vi "Transmit CAN.vi"(0 "CAN Queue":T1, 2 "CAN frame":T2 {"type" items=["CAN Data", "CAN Remote"]; "identifier" format="%.0x"}) -> (7 "CAN Queue Out":T1)   [LabVIEW 2014]
uses:
  <vilib>/RioEmbeddedCAN/RioEmbeddedCAN.llb/CANFrameControl.ctl
  CAN Message Queue.ctl
  CAN Message.ctl
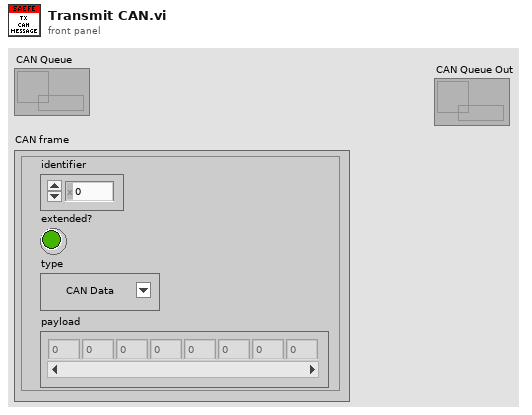
[diagram p1: front panel]
types:
  T1 = typedef "CAN Message Queue.ctl" = refnum<k33>
  T2 = typedef "CANFrameControl.ctl" = cluster{"identifier":u32, "extended?":bool, "type":u8, "payload":u8[]}
  T3 = cluster{"B0":u8, "B1":u8, "B2":u8, "B3":u8, "B4":u8, "B5":u8, "B6":u8, "B7":u8}
  T4 = typedef "CAN Message.ctl" = cluster{"identifier":u32, "extended?":bool, "type":u8, "data":cluster{"B0":u8, "B1":u8, "B2":u8, "B3":u8, "B4":u8, "B5":u8, "B6":u8, "B7":u8}}
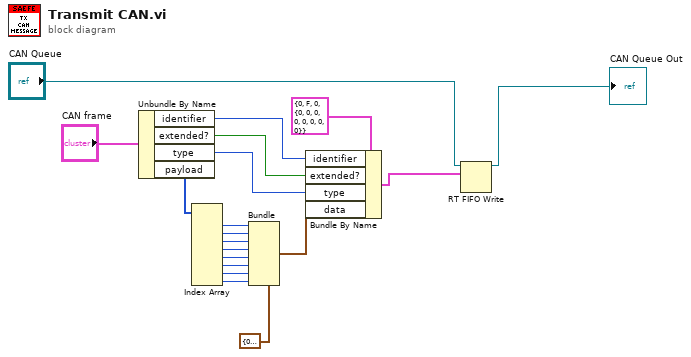
[diagram p0: block diagram]
diagram:
  n1 = Unbundle By Name("CAN frame") -> ("identifier"=w15:u32, "extended?"=w14:bool, "type"=w13:u8, "payload"=w12:u8[])
  n2 = Index Array(array=w12) -> (element #1=w11:u8, element #2=w10:u8, element #3=w9:u8, element #4=w8:u8, element #5=w7:u8, element #6=w6:u8, element #7=w5:u8, element #8=w4:u8)  [unwired: 8 in]
  n3 = Bundle(cluster=T3 {"B0"=0, "B1"=0, "B2"=0, "B3"=0, "B4"=0, "B5"=0, "B6"=0, "B7"=0} ("data"), "B0"=w11, "B1"=w10, "B2"=w9, "B3"=w8, "B4"=w7, "B5"=w6, "B6"=w5, "B7"=w4) -> (w16:T3)
  n4 = Bundle By Name(cluster=T4 {"identifier"=0, "extended?"=FALSE, "type"=0, "data"={"B0"=0, "B1"=0, "B2"=0, "B3"=0, "B4"=0, "B5"=0, "B6"=0, "B7"=0}} ("CAN frame"), "identifier"=w15, "extended?"=w14, "type"=w13, "data"=w16) -> (w1:T4)
  n5 = RT FIFO Write(0:"CAN Queue", 1:w1) -> (8:→"CAN Queue Out":T1)  [unwired: 3 in, 3 out]
